vi "DriveOutput.vi"   [LabVIEW 2017]
uses:
  DriveOutput.ctl
  <vilib>/Rock Robotics/WPI/ThirdParty/Phoenix-LabVIEW/Motor Controller/Controls/CTRE_Phoenix_MotorControl_ControlMode.ctl
  SubsystemData/DriveData/DriveData.lvclass
types:
  T1 = typedef "DriveData.lvclass/DriveOutput.ctl" = cluster{"LeftDriveSetting":dbl, "RightDriveSetting":dbl, "Control Mode":T2}
  T2 = typedef "CTRE_Phoenix_MotorControl_ControlMode.ctl" = u16
  T3 = typedef "WPI_MotorControlDeviceRef.ctl" = cluster{"DeviceStatus":errorcluster, "Type":T4, "PWM":cluster{"PWM Channel":T5, "DeadBand":T6}, "CAN":cluster{"Device Number":u8, "SetOutput VI Ref":variant, "GetOutput VI Ref":variant, "Enable VI Ref":variant, "Disable VI Ref":variant, "Data":variant}, "Invert":bool, "DIO PWM":cluster{"PWM \"Enable\" Channel":T5, "DIOChannel":T7, "PWM Rate":dbl}}
  T4 = typedef "WPI_MotorControlType.ctl" = enum16{"PWM", "CAN", "DIO PWM"}
  T5 = typedef "FPGA_DIOPWMChannel.ctl" = enum8{"PWM 0", "PWM 1", "PWM 2", "PWM 3", "PWM 4", "PWM 5", "PWM 6", "PWM 7", "PWM 8", "PWM 9", "PWM MXP 0", "PWM MXP 1", "PWM MXP 2", "PWM MXP 3", "PWM MXP 4", "PWM MXP 5", "PWM MXP 6", "PWM MXP 7", "PWM MXP 8", "PWM MXP 9", "Invalid"}
  T6 = typedef "WPI_PWMDeadband.ctl" = cluster{"Name":string, "maxPositivePwm":i32, "minPositivePwm":i32, "centerPwm":i32, "maxNegativePwm":i32, "minNegativePwm":i32, "angularRange":u16}
  T7 = typedef "FPGA_DIOChannel.ctl" = enum8{"DIO 0", "DIO 1", "DIO 2", "DIO 3", "DIO 4", "DIO 5", "DIO 6", "DIO 7", "DIO 8", "DIO 9", "DIO MXP 0", "DIO MXP 1", "DIO MXP 2", "DIO MXP 3", "DIO MXP 4", "DIO MXP 5", "DIO MXP 6", "DIO MXP 7", "DIO MXP 8", "DIO MXP 9", "DIO MXP 10", "DIO MXP 11", "DIO MXP 12", "DIO MXP 13", "DIO MXP 14", "DIO MXP 15", "SPI Port CS1", "SPI Port CS2", "SPI Port CS3", "SPI Port MISO", "SPI Port MOSI", "Invalid"}
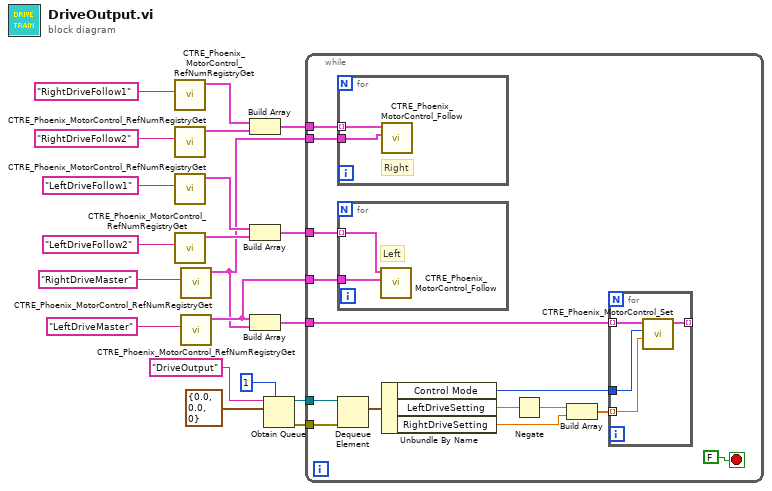
[diagram p0: block diagram]
diagram:
  n1 = call <vilib>:"CTRE_Phoenix_MotorControl_RefNumRegistryGet.vi"("refnum name"="RightDriveFollow1") -> ("PhoenixMotorControlDevRef"=w12:T3)  [unwired: 9 in, 1 out]
  n2 = call <vilib>:"CTRE_Phoenix_MotorControl_RefNumRegistryGet.vi"("refnum name"="RightDriveFollow2") -> ("PhoenixMotorControlDevRef"=w8:T3)  [unwired: 9 in, 1 out]
  n3 = call <vilib>:"CTRE_Phoenix_MotorControl_RefNumRegistryGet.vi"("refnum name"="LeftDriveFollow1") -> ("PhoenixMotorControlDevRef"=w4:T3)  [unwired: 9 in, 1 out]
  n4 = call <vilib>:"CTRE_Phoenix_MotorControl_RefNumRegistryGet.vi"("refnum name"="LeftDriveFollow2") -> ("PhoenixMotorControlDevRef"=w7:T3)  [unwired: 9 in, 1 out]
  n5 = call <vilib>:"CTRE_Phoenix_MotorControl_RefNumRegistryGet.vi"("refnum name"="RightDriveMaster") -> ("PhoenixMotorControlDevRef"=w1:T3)  [unwired: 9 in, 1 out]
  n6 = call <vilib>:"CTRE_Phoenix_MotorControl_RefNumRegistryGet.vi"("refnum name"="LeftDriveMaster") -> ("PhoenixMotorControlDevRef"=w2:T3)  [unwired: 9 in, 1 out]
  n7 = Build Array(w12, w8) -> (w10:T3[])
  n8 = Build Array(w4, w7) -> (w3:T3[])
  n9 = Build Array(w2, w1) -> (w13:T3[])
  n10 = Obtain Queue(max queue size (-1, unlimited)=1, name (unnamed)="DriveOutput", element data type=T1 {"LeftDriveSetting"=0.0, "RightDriveSetting"=0.0, "Control Mode"=0} ("DriveOutput")) -> (queue out=w19:refnum<queue>, error out=w20:errorcluster)  [unwired: 2 in, 1 out]
  n11 = while {
    tunnel: w20 -> [w32]
    tunnel: w19 -> [w31]
    tunnel: w13 -> [w26]
    tunnel: w10 -> [w25]
    tunnel: w3 -> [w24]
    tunnel: w2 -> [w23]
    tunnel: w1 -> [w22]
    stop <- FALSE stop-if-true
    n12 = for {
      tunnel: w25 -> [w38] mode=indexing
      tunnel: w22 -> [w37]
      # "Right"
      n13 = call <vilib>:"CTRE_Phoenix_MotorControl_Follow.vi"("Master Controller to Follow"=w37, "PhoenixMotorControlDevRef"=w38) -> ()  [unwired: 8 in, 2 out]
    }
    n14 = for {
      tunnel: w24 -> [w36] mode=indexing
      tunnel: w23 -> [w35]
      # "Left"
      n15 = call <vilib>:"CTRE_Phoenix_MotorControl_Follow.vi"("Master Controller to Follow"=w35, "PhoenixMotorControlDevRef"=w36) -> ()  [unwired: 8 in, 2 out]
    }
    n16 = Dequeue Element(queue=w31, error in (no error)=w32) -> (element=w33:T1)  [unwired: 1 in, 3 out]
    n17 = Unbundle By Name(w33) -> ("Control Mode"=w27:T2, "LeftDriveSetting"=w29:dbl, "RightDriveSetting"=w28:dbl)
    n18 = Negate(x=w29) -> (-x=w21:dbl)
    n19 = Build Array(w21, w28) -> (w34:dbl[])
    n20 = for {
      tunnel: w27 -> [w42]
      tunnel: w34 -> [w41] mode=indexing
      tunnel: [w40] -> _ mode=indexing
      tunnel: w26 -> [w39] mode=indexing
      n21 = call <vilib>:"CTRE_Phoenix_MotorControl_Set.vi"("Output"=w41, "Control Mode"=w42, "PhoenixMotorControlDevRef"=w39) -> ("PhoenixMotorControlDevRef"=w40:T3)  [unwired: 7 in, 1 out]
    }
  }
